vi "Log.Litho.Playground.vi"() -> ()   [LabVIEW 2019, in "Log.Litho.lvclass"]
uses:
  Log.Litho.lvclass
  <vilib>/Utility/sysdir.llb/Get System Directory.vi
panel:
  out "String":string
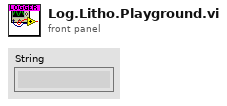
[diagram p1: front panel]
types:
  T1 = enum16{"open", "replace", "create", "open or create", "replace or create", "replace or create with confirmation"}
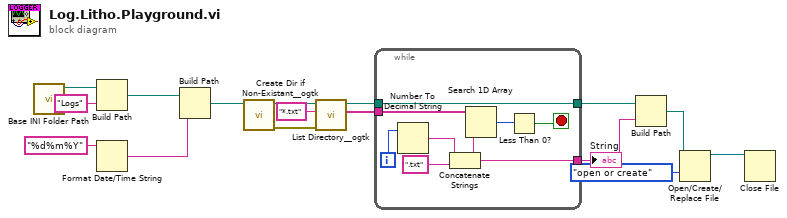
[diagram p0: block diagram]
diagram:
  n1 = call "Base INI Folder Path.vi"() -> ("Base Path"=w16:path)  [unwired: 11 in]
  n2 = Build Path(base path=w16, name or relative path="Logs") -> (appended path=w14:path)
  n3 = Format Date/Time String(time format string (%c)="%d%m%Y") -> (date/time string=w12:string)  [unwired: 2 in]
  n4 = Build Path(base path=w14, name or relative path=w12) -> (appended path=w11:path)
  n5 = call <userlib>:"Create Dir if Non-Existant__ogtk.vi"("Directory Path"=w11) -> ("error out"=w8:errorcluster, "dup Directory Path"=w10:path)  [unwired: 8 in, 1 out]
  n6 = call <userlib>:"List Directory__ogtk.vi"("error in (no error)"=w8, "pattern"="*.txt", "directory path"=w10) -> ("file names"=w7:string[], "dup directory path"=w5:path)  [unwired: 1 in, 2 out]
  n7 = while {
    tunnel: w7 -> [w24]
    tunnel: [w19] -> w4
    tunnel: [w17] -> w6
    tunnel: w5 -> [w17]
    i -> [w23]
    stop <- w18 stop-if-true
    n8 = Number To Decimal String(number=w23) -> (decimal integer string=w20:string)  [unwired: 1 in]
    n9 = Concatenate Strings(w20, ".txt" ("string")) -> (w19:string)
    n10 = Search 1D Array(1D array=w24, element=w19) -> (index of element=w22:i32)  [unwired: 1 in]
    n11 = Less Than 0?(x=w22) -> (x < 0?=w18:bool)
  }
  "String" <- w4
  n12 = Build Path(base path=w6, name or relative path=w4) -> (appended path=w3:path)
  n13 = Open/Create/Replace File(file path (use dialog)=w3, operation (0:open)=T1."open or create") -> (refnum out=w2:refnum<file>)  [unwired: 4 in, 2 out]
  n14 = Close File(refnum=w2) -> ()  [unwired: 1 in, 2 out]
